vi "Status.vi"(3 "error in (no error)":errorcluster, 4 "Output channel":T1, 5 "VISA resource name":refnum<visa-resource-name>) -> (0 "error out":errorcluster, 1 "Status identifier":string, 2 "VISA resource name out":refnum<visa-resource-name>)   [LabVIEW 2014, in "YbTempCtrl.lvlib"]
doc: "Get a string representing the current state of the controller"
uses:
  YbTempCtrl.lvlib
  Typedefs/OutputChannelTypedef.ctl
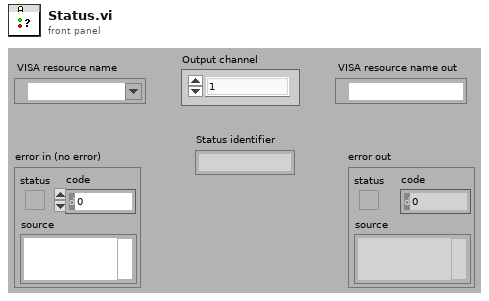
[diagram p1: front panel]
types:
  T1 = typedef "YbTempCtrl.lvlib/OutputChannelTypedef.ctl" = enum16{"1", "2", "BP"}
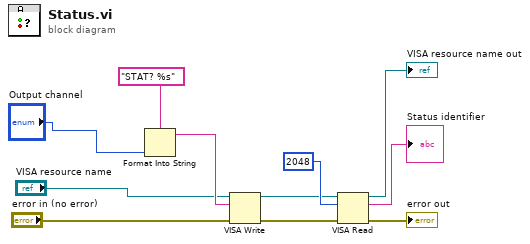
[diagram p0: block diagram]
diagram:
  n1 = Format Into String(format string="STAT? %s" ("write buffer"), "Output channel") -> (resulting string=w5:string)  [unwired: 2 in, 1 out]
  n2 = VISA Write(VISA resource name="VISA resource name", write buffer=w5, error in (no error)="error in (no error)") -> (VISA resource name out=w7:refnum<visa-resource-name>, error out=w6:errorcluster)  [unwired: 1 out]
  n3 = VISA Read(VISA resource name=w7, byte count=u32 2048, error in (no error)=w6) -> (VISA resource name out=→"VISA resource name out":refnum<visa-resource-name>, read buffer=→"Status identifier":string, error out=→"error out":errorcluster)  [unwired: 1 out]
